vi "Close Log File.vi"(6 "MinMax_in":dbl[][](array[numeric]), 8 "error in (no error)":errorcluster, 10 "Data Queue":refnum<queue>, 11 "Logging Configuration":T1={"Log File Base Path"=path "", "Samples to Save"=0, "Trigger - Threshold"=0.0, "Trigger - Channel"=0, "Always Log"=FALSE, "External Trigger"=FALSE, "External Trigger Armed"=FALSE, "TDMS File Reference"=refnum, "DAQVersion"="", "SWVersion"="", "CircSamples"=0, "BeepWhenComplete"=FALSE, "ChannelConfig"=[], "ActiveChannels"=[], "Title"="", "Description"="", "ChannelNames"=[], "ResponseExtension"=TRUE}) -> (0 "error out":errorcluster)   [LabVIEW 2017, in "Logging.lvlib"]
doc: "Flush the data queue of any pending data and write it to the log file. Close the TDMS file reference."
uses:
  Logging.lvlib
  Logging Configuration.ctl
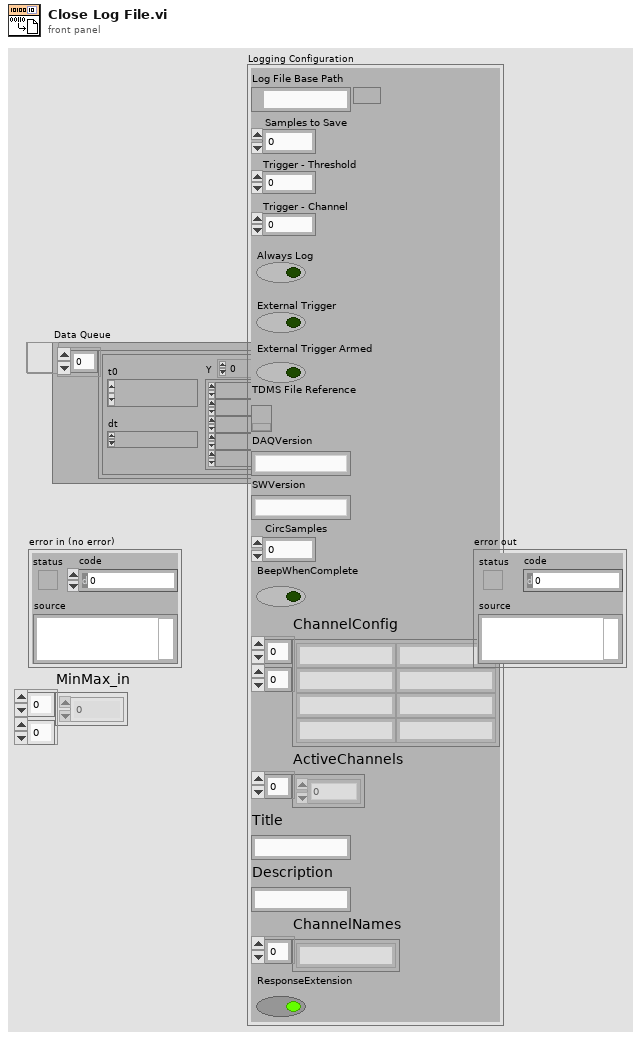
[diagram p1: front panel]
types:
  T1 = typedef "Logging.lvlib/Logging Configuration.ctl" = cluster{"Log File Base Path":path, "Samples to Save":u32, "Trigger - Threshold":dbl, "Trigger - Channel":u32, "Always Log":bool, "External Trigger":bool, "External Trigger Armed":bool, "TDMS File Reference":refnum<k34>, "DAQVersion":string, "SWVersion":string, "CircSamples":u32, "BeepWhenComplete":bool, "ChannelConfig":string[][], "ActiveChannels":i32[], "Title":string, "Description":string, "ChannelNames":string[], "ResponseExtension":bool}
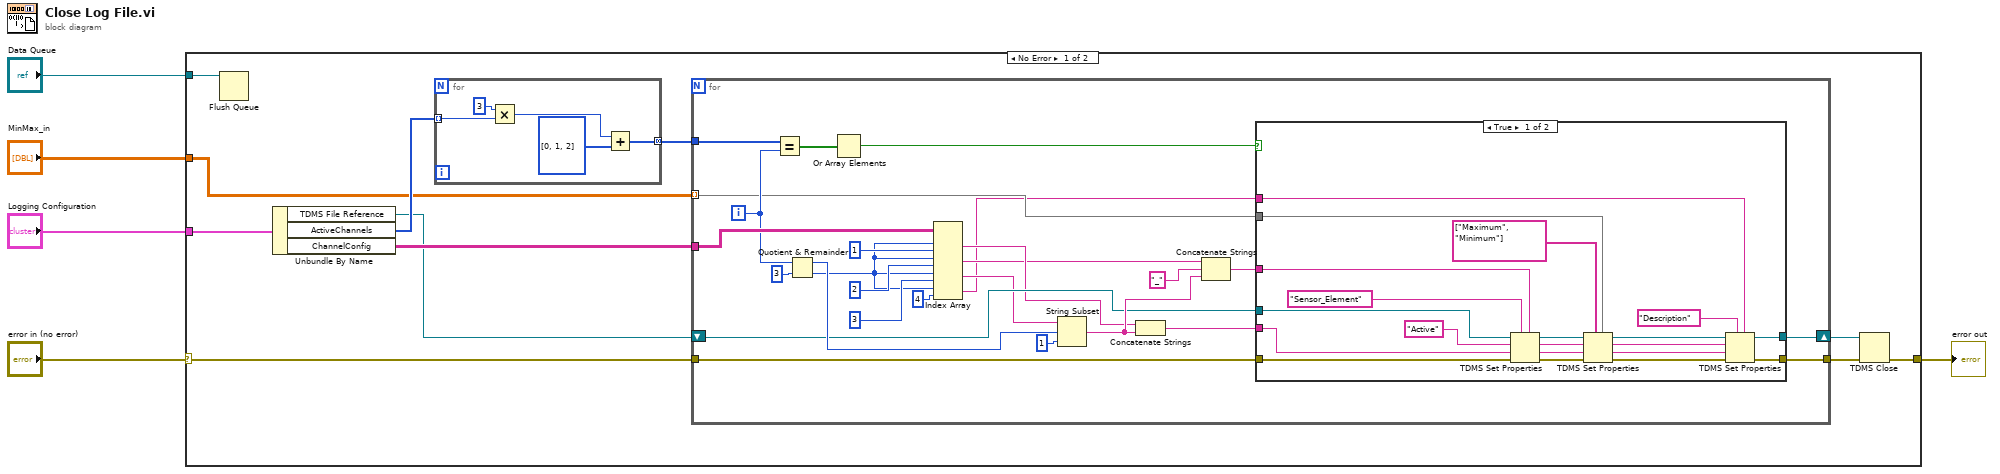
[diagram p0: block diagram]
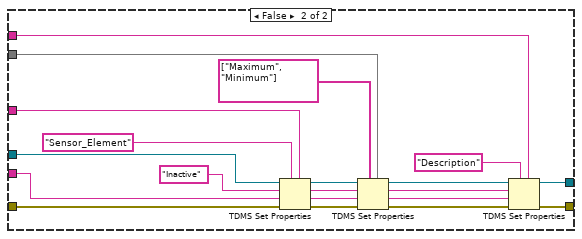
[diagram p2: hidden frame]
diagram:
  n1 = case shown="No Error" "error in (no error)" {
    selector: "error in (no error)" -> [w10 w88]
    tunnel: "Data Queue" -> [w16 _]
    tunnel: "Logging Configuration" -> [w15 _]
    tunnel: "MinMax_in" -> [w12 _]
    tunnel: [w6 w88] -> w1
    frame No Error {
      n2 = Flush Queue(queue=w16) -> ()  [unwired: 1 in, 3 out]
      n3 = Unbundle By Name(w15) -> ("TDMS File Reference"=w7:refnum<k34>, "ActiveChannels"=w14:i32[], "ChannelConfig"=w13:string[][])
      n4 = for {
        tunnel: w14 -> [w87] mode=indexing
        tunnel: [w83] -> w11 mode=concatenating
        n5 = Multiply(x=3, y=w87) -> (x*y=w85:i32)
        n6 = Add(x=w85, y=i32[] [0, 1, 2]) -> (x+y=w83:i32[])
      }
      n7 = for {
        tunnel: w12 -> [w26] mode=indexing
        tunnel: w11 -> [w42]
        tunnel: w13 -> [w39]
        tunnel: w10 -> [w30]
        tunnel: [w29] -> w9
        shift-right: [w28] -> w8
        shift-left: w7 -> [w24]
        i -> [w34]
        n8 = Equal?(x=w42, y=w34) -> (x = y?=w41:bool[])
        n9 = Quotient & Remainder(x=w34, y=3) -> (x-y*floor(x/y)=w40:i32, floor(x/y)=w18:i32)
        n10 = Or Array Elements(Boolean array=w41) -> (logical OR=w31:bool)
        n11 = Index Array(array=w39, index (row) #1=w18, index (col) #1=1 ("disabled index (col)"), index (row) #2=w18, index (col) #2=2 ("disabled index (col)"), index (row) #3=w18, index (col) #3=3 ("index (col)"), index (row) #4=w18, index (col) #4=4 ("index (col)")) -> (element #1=w22:string, element #2=w20:string, element #3=w21:string, element #4=w17:string)
        n12 = String Subset(string=w21, offset (0)=w40, length (rest)=1 ("length (rest)")) -> (substring=w32:string)
        n13 = Concatenate Strings(w22, w32) -> (w27:string)
        n14 = Concatenate Strings(w20, "_" ("string"), w32) -> (w25:string)
        n15 = case shown="True" w31 {
          tunnel: w30 -> [w56 w76]
          tunnel: w24 -> [w54 w74]
          tunnel: [w47 w65] -> w29
          tunnel: [w48 w66] -> w28
          tunnel: w27 -> [w53 w73]
          tunnel: w26 -> [w51 w71]
          tunnel: w25 -> [w52 w72]
          tunnel: w17 -> [w43 w69]
          frame True {
            n16 = TDMS Set Properties(5:w52, 7:"Sensor_Element" ("name"), 8:w56, 9:w53, 10:"Active" ("t"), 11:w54) -> (0:w61:errorcluster, 1:w59:string, 2:w60:string, 3:w62:refnum<k34>)
            n17 = TDMS Set Properties(5:w51, 7:string[] ["Maximum", "Minimum"] ("property names"), 8:w61, 9:w59, 10:w60, 11:w62) -> (0:w50:errorcluster, 1:w45:string, 2:w46:string, 3:w49:refnum<k34>)
            n18 = TDMS Set Properties(5:w43, 7:"Description" ("name"), 8:w50, 9:w45, 10:w46, 11:w49) -> (0:w47:errorcluster, 3:w48:refnum<k34>)  [unwired: 2 out]
          }
          frame False {
            n19 = TDMS Set Properties(5:w72, 7:"Sensor_Element" ("name"), 8:w76, 9:w73, 10:"Inactive" ("t"), 11:w74) -> (0:w81:errorcluster, 1:w79:string, 2:w80:string, 3:w82:refnum<k34>)
            n20 = TDMS Set Properties(5:w71, 7:string[] ["Maximum", "Minimum"] ("property names"), 8:w81, 9:w79, 10:w80, 11:w82) -> (0:w68:errorcluster, 1:w63:string, 2:w64:string, 3:w67:refnum<k34>)
            n21 = TDMS Set Properties(5:w69, 7:"Description" ("name"), 8:w68, 9:w63, 10:w64, 11:w67) -> (0:w65:errorcluster, 3:w66:refnum<k34>)  [unwired: 2 out]
          }
        }
      }
      n22 = TDMS Close(8:w9, 11:w8) -> (0:w6:errorcluster)  [unwired: 1 out]
    }
    frame Error {
    }
  }
  "error out" <- w1
